vi "clfilereader_readStr.vi"(9 "size":u32, 10 "offset":u32, 11 "clFileReader.lvclass IN":refnum<class "clFileReader.lvclass">) -> (0 "ReadStr - OUT Value":string, 1 "EOF?":bool, 2 "new offset":u32, 3 "clFileReader.lvclass OUT":refnum<class "clFileReader.lvclass">)   [LabVIEW 2020, in "vi_lib.lvlib" / "clFileReader.lvclass"]
uses:
  clFileReader.lvclass
  clFileReader.lvclass/clFileReader.ctl
  clFile/clFile.lvclass
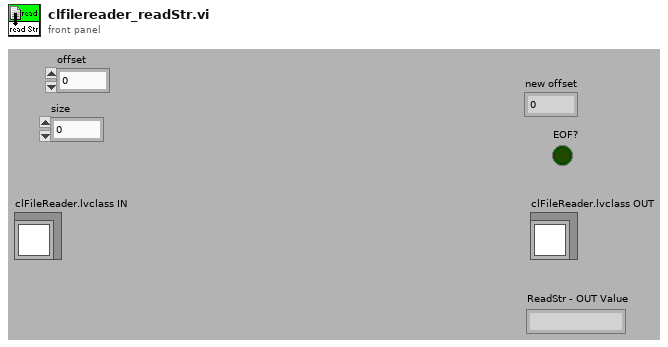
[diagram p1: front panel]
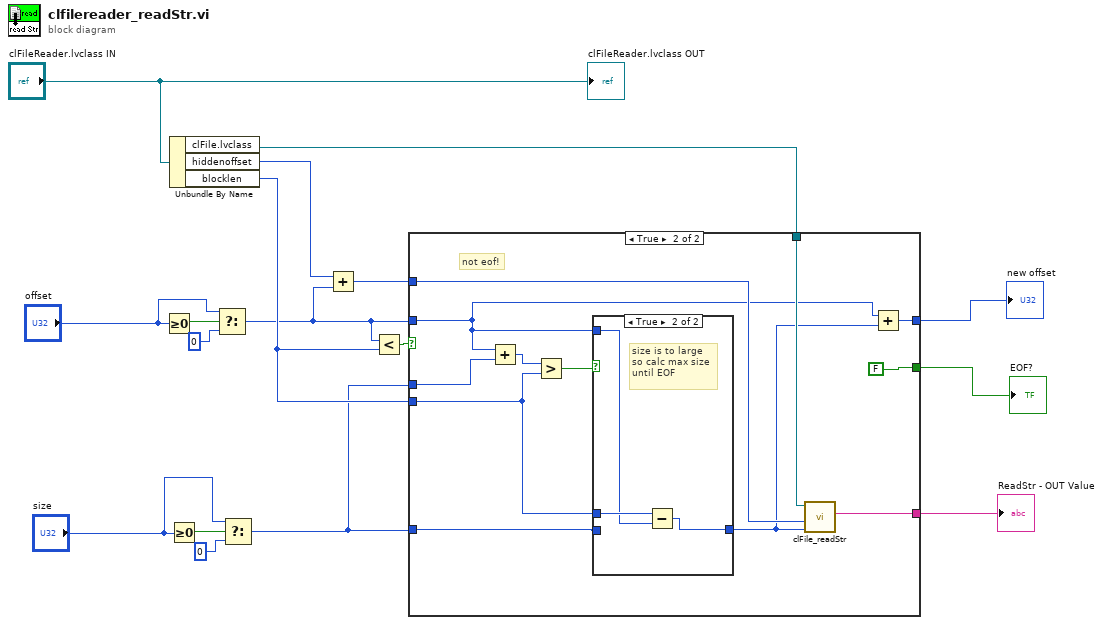
[diagram p0: block diagram]
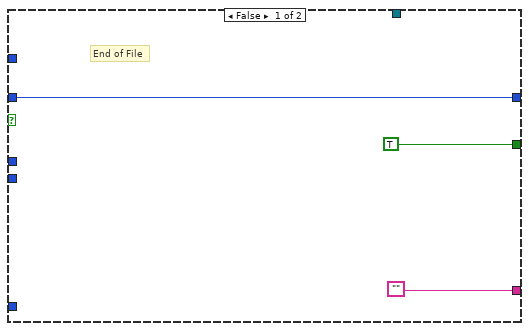
[diagram p2: hidden frame]
diagram:
  n1 = Greater Or Equal To 0?(x="offset") -> (x >= 0?=w13:bool)
  n2 = Greater Or Equal To 0?(x="size") -> (x >= 0?=w16:bool)
  n3 = Unbundle By Name("clFileReader.lvclass IN") -> ("clFile.lvclass"=w5:refnum<class "clFile.lvclass">, "hiddenoffset"=w10:u32, "blocklen"=w8:u32)
  n4 = Select(t="offset", s=w13, f=u32 0) -> (s? t:f=w2:u32)
  n5 = Select(t="size", s=w16, f=u32 0) -> (s? t:f=w6:u32)
  n6 = Add(x=w10, y=w2) -> (x+y=w1:u32)
  n7 = Less?(x=w2, y=w8) -> (x < y?=w9:bool)
  n8 = case shown="True" w9 {
    tunnel: w2 -> [w19 w22]
    tunnel: w6 -> [_ w32]
    tunnel: w8 -> [_ w28]
    tunnel: [TRUE ("EOF?") FALSE ("EOF?")] -> w7
    tunnel: w6 -> [_ w29]
    tunnel: w5 -> [_ w27]
    tunnel: w1 -> [_ w26]
    tunnel: ["" w25] -> w4
    tunnel: [w19 w23] -> w3
    frame False {
      # "End of File"
    }
    frame True {
      # "not eof!"
      n9 = Add(x=w22, y=w32) -> (x+y=w31:u32)
      n10 = Greater?(x=w31, y=w28) -> (0:w30:bool)
      n11 = case shown="True" w30 {
        tunnel: w29 -> [w33 _]
        tunnel: w28 -> [_ w36]
        tunnel: w22 -> [_ w35]
        tunnel: [w33 w34] -> w21
        frame False {
        }
        frame True {
          # "size is to large\nso calc max size\nuntil EOF"
          n12 = Subtract(x=w36, y=w35) -> (x-y=w34:u32)
        }
      }
      n13 = call "clFile_readStr.vi"("length"=w21, "offset (0)"=w26, "clFile.lvclass"=w27) -> ("substring"=w25:string)  [unwired: 7 out]
      n14 = Add(x=w22, y=w21) -> (x+y=w23:u32)
    }
  }
  "new offset" <- w3
  "EOF?" <- w7
  "ReadStr - OUT Value" <- w4
  "clFileReader.lvclass OUT" <- "clFileReader.lvclass IN"
